vi "Open_Instr.vi"(8 "error in (no error)":errorcluster caption="entrée d'erreur (pas d'erreur)", 11 "Class DIO en entrée":refnum<class "Class Instrument Log_File.lvclass">) -> (0 "error out":errorcluster caption="sortie d'erreur", 3 "Class DIO en Sortie":refnum<class "Class Instrument Log_File.lvclass">)   [LabVIEW 2020, in "Library Instrument & Equipement.lvlib" / "Library Instruments.lvlib" / "Class Instrument Log_File.lvclass"]
uses:
  Class Instrument Log_File.lvclass
  Read CSV File/CSV_File (Default)/Class CSV_File.lvclass
  C:/Users/ngarcin/OneDrive - Altyor/Standard TB/Class/Read CSV File/Class File (Default)/Class File (Default).lvclass
  Class Instrument Log_File.lvclass/Class Instrument Log_File.ctl
  Log File/Class Log_File Altyor/Class Log_File Altyor.lvclass
  C:/Users/ngarcin/OneDrive - Altyor/Standard TB/Class/Log File/Log_File (Default)/Class Log_File (Default).lvclass
  Instrument (Default)/Class Instrument (Default).lvclass
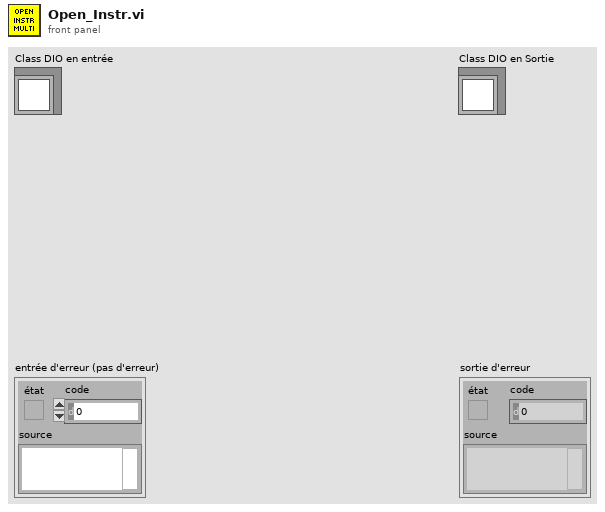
[diagram p1: front panel]
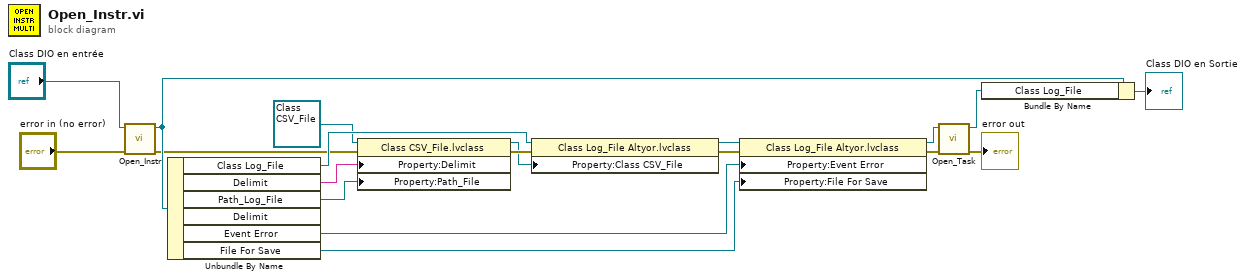
[diagram p0: block diagram]
diagram:
  n1 = call-parent "Open_Instr.vi"("error in (no error)"="error in (no error)", "Class Multimeter (Default) en entrée"="Class DIO en entrée") -> ("error out"=w12:errorcluster, "Class Multimeter (Default) en sortie"=w16:refnum<class "Class Instrument Log_File.lvclass">)  [unwired: 8 in]
  n2 = Unbundle By Name(w16) -> ("Class Log_File"=w17:refnum<class "Class Log_File Altyor.lvclass">, "Delimit"=w8:string, "Path_Log_File"=w7:path, "Event Error"=w2:refnum<user-event>, "File For Save"=w1:refnum<queue>)  [unwired: 1 out]
  n3 = property class="Class CSV_File.lvclass"(reference=refnum<class "Class CSV_File.lvclass"> refnum ("Library File.lvlib:Class CSV_File.lvclass"), error in=w12, "Property:Delimit"=w8, "Property:Path_File"=w7) -> (reference out=w9:refnum<class "Class CSV_File.lvclass">, error out=w10:errorcluster)
  n4 = property class="Class Log_File Altyor.lvclass"(reference=w17, error in=w10, "Property:Class CSV_File"=w9) -> (reference out=w6:refnum<class "Class Log_File Altyor.lvclass">, error out=w5:errorcluster)
  n5 = property class="Class Log_File Altyor.lvclass"(reference=w6, error in=w5, "Property:Event Error"=w2, "Property:File For Save"=w1) -> (reference out=w3:refnum<class "Class Log_File Altyor.lvclass">, error out=w4:errorcluster)
  n6 = call-dynamic "Open_Task.vi"("error in (no error)"=w4, "Class Log_File Altyor en entrée"=w3) -> ("error out"=→"error out":errorcluster, "Class Log_File Altyor en sortie"=w13:refnum<class "Class Log_File Altyor.lvclass">)  [unwired: 8 in]
  n7 = Bundle By Name(cluster=w16, "Class Log_File"=w13) -> (→"Class DIO en Sortie":refnum<class "Class Instrument Log_File.lvclass">)
